vi "oax_gsGet Next Events.vi"(0 "event queue in":string[](array[string])) -> (1 "next event":string, 2 "event queue out":string[](array[string]))   [LabVIEW 2017]
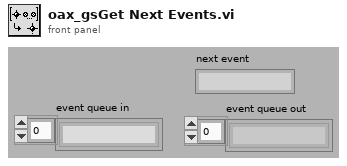
[diagram p1: front panel]
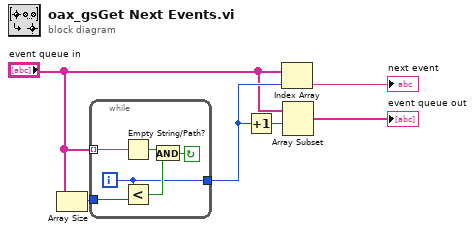
[diagram p0: block diagram]
diagram:
  n1 = Array Size(array="event queue in") -> (size(s)=w5:i32)
  n2 = while {
    tunnel: "event queue in" -> [w12] mode=indexing
    tunnel: w5 -> [w11]
    tunnel: [w7] -> w4
    i -> [w7]
    stop <- w8 continue-if-true
    n3 = Empty String/Path?(string/path=w12) -> (empty?=w10:bool)
    n4 = Less?(x=w7, y=w11) -> (x < y?=w9:bool)
    n5 = And(x=w10, y=w9) -> (x .and. y?=w8:bool)
  }
  n6 = Increment(x=w4) -> (x+1=w6:i32)
  n7 = Index Array(array="event queue in", index=w4) -> (element=→"next event":string)
  n8 = Array Subset(array="event queue in", index=w6) -> (→"event queue out":string[])  [unwired: 1 in]
